vi "Basic Print Test.vi"() -> ()   [LabVIEW 2014, in "ESP8266 WiFi Wrapper.lvlib"]
uses:
  <vilib>/Aledyne-TSXperts/Arduino Compatible Compiler for LabVIEW/addons/ESP8266 WiFi Wrapper/ESP8266 WiFi Wrapper.lvlib
panel:
  out "Error Out":errorcluster
  in  "Error In":errorcluster
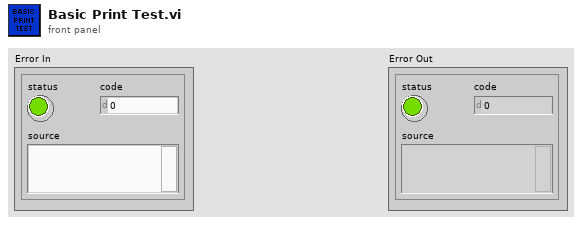
[diagram p1: front panel]
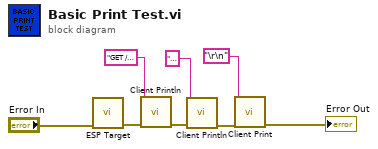
[diagram p0: block diagram]
diagram:
  n1 = call <vilib>:"ESP Target.vi"("Error In"="Error In") -> ("Error Out"=w2:errorcluster)  [unwired: 10 in]
  n2 = call <vilib>:"Client Println.vi"("Error In"=w2, "Input String"="GET /hello HTTP/1.0") -> ("Error Out"=w7:errorcluster)  [unwired: 9 in]
  n3 = call <vilib>:"Client Println.vi"("Error In"=w7, "Input String"="Connection: close") -> ("Error Out"=w5:errorcluster)  [unwired: 9 in]
  n4 = call <vilib>:"Client Print.vi"("Error In"=w5, "Input String"="\r\n") -> ("Error Out"=→"Error Out":errorcluster)  [unwired: 9 in]
